vi "scale-wisher-sorter.vi"(11 "Scales":T1) -> (3 "Scale notes":bool[](array[boolean]))   [LabVIEW 2019]
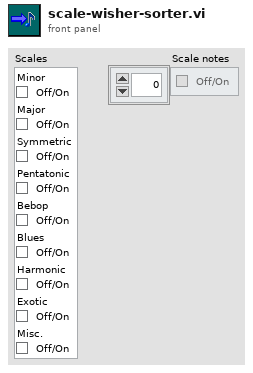
[diagram p1: front panel]
types:
  T1 = cluster{"Minor":bool, "Major":bool, "Symmetric":bool, "Pentatonic":bool, "Bebop":bool, "Blues":bool, "Harmonic":bool, "Exotic":bool, "Misc.":bool}
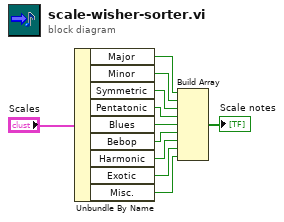
[diagram p0: block diagram]
diagram:
  n1 = Unbundle By Name("Scales") -> ("Major"=w2:bool, "Minor"=w3:bool, "Symmetric"=w4:bool, "Pentatonic"=w5:bool, "Blues"=w6:bool, "Bebop"=w7:bool, "Harmonic"=w8:bool, "Exotic"=w9:bool, "Misc."=w10:bool)
  n2 = Build Array(w2, w3, w4, w5, w6, w7, w8, w9, w10) -> (→"Scale notes":bool[])
